vi "DestroyClone.vi"(8 "error in (no error)":errorcluster, 9 "Exit via Stop Module Req?":bool, 10 "Wait for Module to stop?":bool, 11 "ModuleAdmin":refnum<class "ModuleAdmin.lvclass">) -> (0 "error out":errorcluster, 1 "External Launch":bool, 3 "Mod Admin out":refnum<class "ModuleAdmin.lvclass">)   [LabVIEW 2018, in "AcPwrPlugins.lvlib"]
doc: "This VI takes care of some cleanup responsibility before allowing Main.vi to close."
uses:
  AcPwrPlugins.lvlib
  <userlib>/NIST/ModuleAdminLib/ModuleAdmin/ModuleAdmin.lvclass
  C:/Program Files (x86)/National Instruments/LabVIEW 2018/user.lib/NIST/ModuleAdminLib/ModuleAdminBase/ModuleAdminBase.lvclass
  <userlib>/NIST/ModuleAdminLib/ModuleAdmin/ModuleAdmin.lvclass/ModuleAdmin.ctl
  <userlib>/NIST/ModuleAdminLib/ModuleAdmin/Accessors/Read CloneRegRef.vi
  <userlib>/NIST/ModuleAdminLib/CloneRegistration/CloneRegistration.lvclass
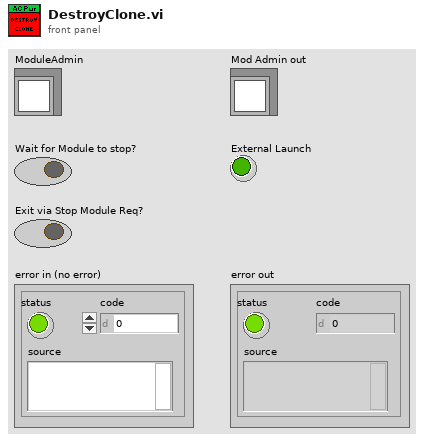
[diagram p1: front panel]
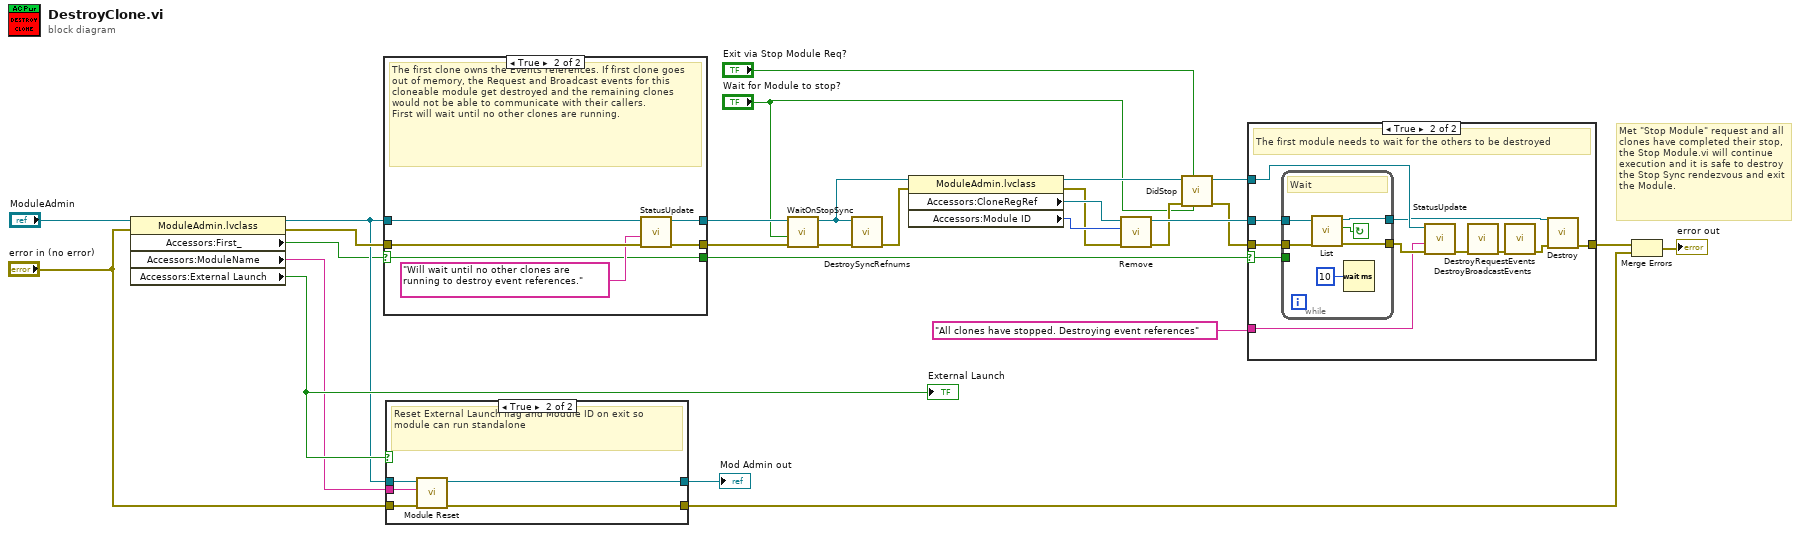
[diagram p0: block diagram]
diagram:
  # "Met \"Stop Module\" request and all clones have completed their stop, the Stop Module.vi will continue execution and it is safe to destroy the Stop Sync rendezvous and exit the Module."
  n1 = property class="ModuleAdmin.lvclass"(reference="ModuleAdmin", error in="error in (no error)") -> (reference out=w5:refnum<class "ModuleAdmin.lvclass">, error out=w13:errorcluster, "Accessors:First_"=w2:bool, "Accessors:ModuleName"=w25:string, "Accessors:External Launch"=w27:bool)
  "External Launch" <- w27
  n2 = case shown="True" w2 {
    selector: w2 -> [w29 w32]
    tunnel: w13 -> [w31 w37]
    tunnel: [w31 w35] -> w17
    tunnel: w5 -> [w30 w34]
    tunnel: [w30 w33] -> w16
    tunnel: [w29 w32] -> w1
    frame False {
    }
    frame True {
      # "The first clone owns the Events references. If first clone goes out of memory, the Request and Broadcast events for this cloneable module get destroyed and the remaining clones would not be able to communicate with their callers.\nFirst will wait until no other clones are running."
      n3 = call "StatusUpdate.vi"("error in (no error)"=w37, "Status"="Will wait until no other clones are running to destroy event references." ("format string"), "Module"=w34) -> ("error out"=w35:errorcluster, "Module"=w33:refnum<class "ModuleAdmin.lvclass">)  [unwired: 7 in]
    }
  }
  n4 = case shown="True" w27 {
    tunnel: "error in (no error)" -> [w38 w44]
    tunnel: w25 -> [_ w43]
    tunnel: w5 -> [w39 w42]
    tunnel: [w39 w41] -> w24
    tunnel: [w38 w40] -> w22
    frame False {
    }
    frame True {
      # "Reset External Launch flag and Module ID on exit so module can run standalone"
      n5 = call <userlib>:"Module Reset.vi"("error in (no error)"=w44, "ModuleName"=w43, "Mod Admin in"=w42) -> ("error out"=w40:errorcluster, "Mod Admin out"=w41:refnum<class "ModuleAdmin.lvclass">)  [unwired: 7 in]
    }
  }
  "Mod Admin out" <- w24
  n6 = call <userlib>:"WaitOnStopSync.vi"("error in (no error)"=w17, "WaitForModuleToStop?"="Wait for Module to stop?", "ModuleAdmin"=w16) -> ("error out"=w28:errorcluster, "ModuleAdmin"=w3:refnum<class "ModuleAdmin.lvclass">)  [unwired: 7 in]
  n7 = call <userlib>:"DestroySyncRefnums.vi"("error in (no error)"=w28, "ModuleAdmin"=w3) -> ("error out"=w15:errorcluster)  [unwired: 9 in]
  n8 = property class="ModuleAdmin.lvclass"(reference=w3, error in=w15) -> (reference out=w11:refnum<class "ModuleAdmin.lvclass">, error out=w14:errorcluster, "Accessors:CloneRegRef"=w20:refnum<data-value>, "Accessors:Module ID"=w19:i32)
  n9 = call <userlib>:"Remove.vi"("error in (no error)"=w14, "Module ID"=w19, "CloneRegRef"=w20) -> ("error out"=w9:errorcluster, "CloneRegRef"=w21:refnum<data-value>)  [unwired: 6 in, 1 out]
  n10 = call "DidStop.vi"("Wait for Module to stop?"="Wait for Module to stop?", "Exit via Stop Module Req?"="Exit via Stop Module Req?", "error in (no error)"=w9, "ModuleAdmin"=w11) -> ("error out"=w8:errorcluster, "ModuleAdmin"=w10:refnum<class "ModuleAdmin.lvclass">)  [unwired: 6 in]
  n11 = case shown="True" w1 {
    selector: w1 -> [_ w55]
    tunnel: w8 -> [w45 w56]
    tunnel: [w45 w49] -> w18
    tunnel: w21 -> [_ w51]
    tunnel: w10 -> [_ w50]
    tunnel: "All clones have stopped. Destroying event references" ("Status") -> [_ w46]
    frame False {
    }
    frame True {
      # "The first module needs to wait for the others to be destroyed"
      n12 = while {
        tunnel: w56 -> [w62]
        tunnel: w55 -> [_]
        tunnel: [w61] -> w54
        tunnel: w51 -> [w58]
        tunnel: [w57] -> w47
        stop <- w60 continue-if-true
        # "Wait"
        n13 = call <userlib>:"List.vi"("error in (no error)"=w62, "CloneRegRef"=w58) -> ("error out"=w61:errorcluster, "Found?"=w60:bool, "CloneRegRef"=w57:refnum<data-value>)  [unwired: 4 in, 3 out]
        n14 = Wait (ms)(milliseconds to wait=u32 10) -> ()  [unwired: 1 out]
      }
      n15 = call "StatusUpdate.vi"("error in (no error)"=w54, "Status"=w46, "Module"=w50) -> ("error out"=w53:errorcluster)  [unwired: 7 in, 1 out]
      n16 = call "DestroyBroadcastEvents.vi"("error in (no error)"=w53) -> ("error out"=w52:errorcluster)  [unwired: 10 in]
      n17 = call "DestroyRequestEvents.vi"("error in (no error)"=w52) -> ("error out"=w48:errorcluster)  [unwired: 10 in]
      n18 = call <userlib>:"Destroy.vi"("error in (no error)"=w48, "CloneRegRef"=w47) -> ("error out"=w49:errorcluster)  [unwired: 9 in]
    }
  }
  n19 = Merge Errors(w18, w22) -> (→"error out":errorcluster)
